vi "xijk_calculate_effective_numbers.vi"(10 "spectra parameters in":T1={"Booleans"={"Unknown detector"=FALSE, "Dual band filters"=FALSE, "Dual emission by cubes"=FALSE, "FRET"=FALSE}, "Integers"={"Light source"=0, "Number of fluorophores"=0, "Wavelength of laser (nm) 1"=0, "Broadness of laser (nm) 1"=0.0, "Wavelength of laser (nm) 2"=0, "Broadness of laser (nm) 2"=0.0, "Template"=1}, "Doubles"={"Molar extinction 1"=1.0, "Molar extinction 2"=1.0, "Quantum efficiency 1"=1.0, "Quantum efficiency 2"=1.0}}, 11 "spectra in":T2) -> (0 "Effective spectral emission 2":sgl[](array[numeric]), 1 "Effective spectral excitation 2":sgl[](array[numeric]), 2 "Effective spectral emission 1":sgl[](array[numeric]), 3 "Effective spectral excitation 1":sgl[](array[numeric]))   [LabVIEW 2010]
uses:
  Type Def/spectrum_table_control.ctl
  Type Def/spectra_parameters.ctl
panel:
  out "Waveform Graph 4":sgl[](graph)
  out "Waveform Graph 3":sgl[](graph)
  out "Waveform Graph 2":sgl[](graph)
  out "Waveform Graph":sgl[](graph)
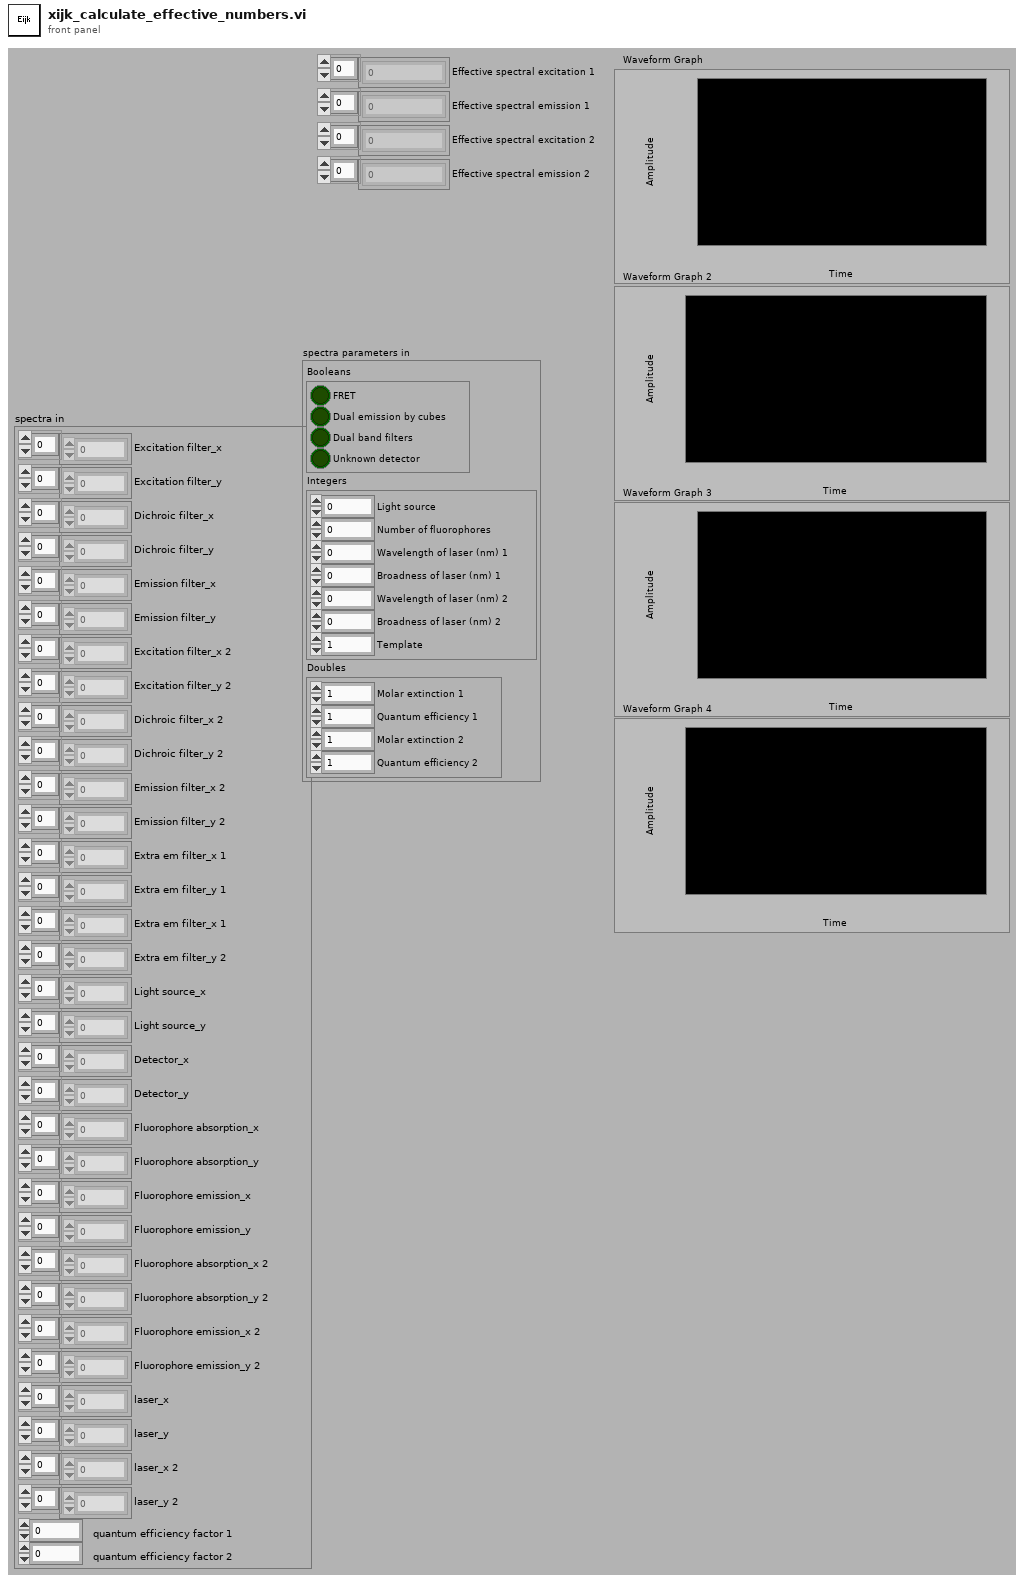
[diagram p1: front panel]
types:
  T1 = typedef "spectra_parameters.ctl" = cluster{"Booleans":cluster{"Unknown detector":bool, "Dual band filters":bool, "Dual emission by cubes":bool, "FRET":bool}, "Integers":cluster{"Light source":u16, "Number of fluorophores":u16, "Wavelength of laser (nm) 1":u16, "Broadness of laser (nm) 1":sgl, "Wavelength of laser (nm) 2":u16, "Broadness of laser (nm) 2":sgl, "Template":u16}, "Doubles":cluster{"Molar extinction 1":sgl, "Molar extinction 2":sgl, "Quantum efficiency 1":sgl, "Quantum efficiency 2":sgl}}
  T2 = typedef "spectrum_table_control.ctl" = cluster{"Excitation filter_x":i16[], "Excitation filter_y":sgl[], "Dichroic filter_x":i16[], "Dichroic filter_y":sgl[], "Emission filter_x":i16[], "Emission filter_y":sgl[], "Excitation filter_x 2":i16[], "Excitation filter_y 2":sgl[], "Dichroic filter_x 2":i16[], "Dichroic filter_y 2":sgl[], "Emission filter_x 2":i16[], "Emission filter_y 2":sgl[], "Extra em filter_x 1":i16[], "Extra em filter_y 1":sgl[], "Extra em filter_x 1":i16[], "Extra em filter_y 2":sgl[], "Light source_x":i16[], "Light source_y":sgl[], "Detector_x":i16[], "Detector_y":sgl[], "Fluorophore absorption_x":i16[], "Fluorophore absorption_y":sgl[], "Fluorophore emission_x":i16[], "Fluorophore emission_y":sgl[], "Fluorophore absorption_x 2":i16[], "Fluorophore absorption_y 2":sgl[], "Fluorophore emission_x 2":i16[], "Fluorophore emission_y 2":sgl[], "laser_x":i16[], "laser_y":sgl[], "laser_x 2":i16[], "laser_y 2":sgl[], "quantum efficiency factor 1":sgl, "quantum efficiency factor 2":sgl}
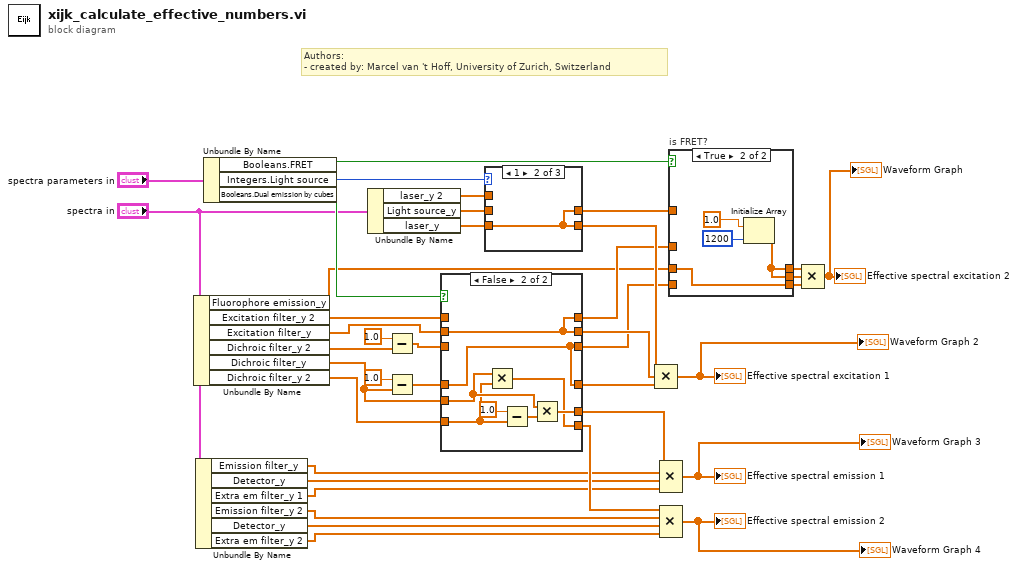
[diagram p0: block diagram]
diagram:
  # "Authors: \n- created by: Marcel van 't Hoff, University of Zurich, Switzerland"
  n1 = Unbundle By Name("spectra in") -> ("Fluorophore emission_y"=w6:sgl[], "Excitation filter_y 2"=w34:sgl[], "Excitation filter_y"=w35:sgl[], "Dichroic filter_y 2"=w36:sgl[], "Dichroic filter_y"=w14:sgl[], "Dichroic filter_y 2"=w13:sgl[])
  n2 = Unbundle By Name("spectra in") -> ("Emission filter_y"=w8:sgl[], "Detector_y"=w9:sgl[], "Extra em filter_y 1"=w10:sgl[], "Emission filter_y 2"=w37:sgl[], "Detector_y"=w11:sgl[], "Extra em filter_y 2"=w12:sgl[])
  n3 = Unbundle By Name("spectra parameters in") -> ("Booleans.FRET"=w17:bool, "Integers.Light source"=w16:u16, "Booleans.Dual emission by cubes"=w15:bool)
  n4 = Unbundle By Name("spectra in") -> ("laser_y 2"=w29:sgl[], "Light source_y"=w31:sgl[], "laser_y"=w30:sgl[])
  n5 = Subtract(x=sgl 1.0, y=w36) -> (x-y=w20:sgl[])
  n6 = Subtract(x=sgl 1.0, y=w14) -> (x-y=w21:sgl[])
  n7 = case shown="False" w15 {
    tunnel: w14 -> [w45 w50]
    tunnel: [w45 w51] -> w39
    tunnel: w13 -> [w44 w49]
    tunnel: [w44 w48] -> w38
    tunnel: w35 -> [w43 w47]
    tunnel: w34 -> [w42 _]
    tunnel: [w43 w47] -> w22
    tunnel: [w42 w47] -> w23
    tunnel: w21 -> [w41 w46]
    tunnel: [w41 w46] -> w19
    tunnel: w20 -> [w40 _]
    tunnel: [w40 w46] -> w18
    frame True {
    }
    frame False {
      n8 = Multiply(x=w50, y=w49) -> (x*y=w48:sgl[])
      n9 = Subtract(x=sgl 1.0, y=w49) -> (x-y=w52:sgl[])
      n10 = Multiply(x=w50, y=w52) -> (x*y=w51:sgl[])
    }
  }
  n11 = case shown="1" w16 {
    tunnel: w30 -> [_ w55 w56]
    tunnel: [w54 w55 w56] -> w33
    tunnel: w31 -> [w54 _ _]
    tunnel: w29 -> [_ _ w57]
    tunnel: [w54 w55 w57] -> w24
    frame 0, Default {
    }
    frame 1 {
    }
    frame 2 {
    }
  }
  n12 = Compound Arithmetic op=MULTIPLY(w33, w22, w19) -> (→"Effective spectral excitation 1" →"Waveform Graph 2":sgl[])
  n13 = Compound Arithmetic op=MULTIPLY(w39, w8, w9, w10) -> (→"Effective spectral emission 1" →"Waveform Graph 3":sgl[])
  n14 = Compound Arithmetic op=MULTIPLY(w38, w37, w11, w12) -> (→"Effective spectral emission 2" →"Waveform Graph 4":sgl[])
  n15 = case "is FRET?" shown="True" w17 {
    tunnel: w23 -> [w60 _]
    tunnel: [w60 w62] -> w26
    tunnel: [w58 w61] -> w25
    tunnel: w24 -> [w59 _]
    tunnel: [w59 w62] -> w32
    tunnel: w18 -> [w58 _]
    tunnel: w6 -> [_ w61]
    frame False {
    }
    frame True {
      n16 = Initialize Array(sgl 1.0 ("élément"), 1200 ("taille de la dimension")) -> (w62:sgl[])
    }
  }
  n17 = Compound Arithmetic op=MULTIPLY(w32, w26, w25) -> (→"Effective spectral excitation 2" →"Waveform Graph":sgl[])
